vi "Lookup by Capabilities.vi"(8 "error in (no error)":errorcluster, 10 "Capabilities":string[](array[string]), 11 "NodeDiscovery in":refnum<class "DiscoveryService.lvclass">) -> (0 "error out":errorcluster, 2 "Nodes":T1[](array[typedef]), 3 "NodeDiscovery out":refnum<class "DiscoveryService.lvclass">)   [LabVIEW 2020, in "Vecto.lvlib" / "DiscoveryService.lvclass"]
uses:
  DiscoveryService.lvclass
  lv-volatus/messages/Discovery/Data.ctl
  lv-volatus/messages/Service/Data.ctl
  lv-volatus/messages/ServiceType/Enumeration.ctl
  lv-volatus/messages/ServiceType/ServiceType.lvlib
  lv-volatus/messages/Service/Service.lvlib
  lv-volatus/messages/Discovery/Discovery.lvlib
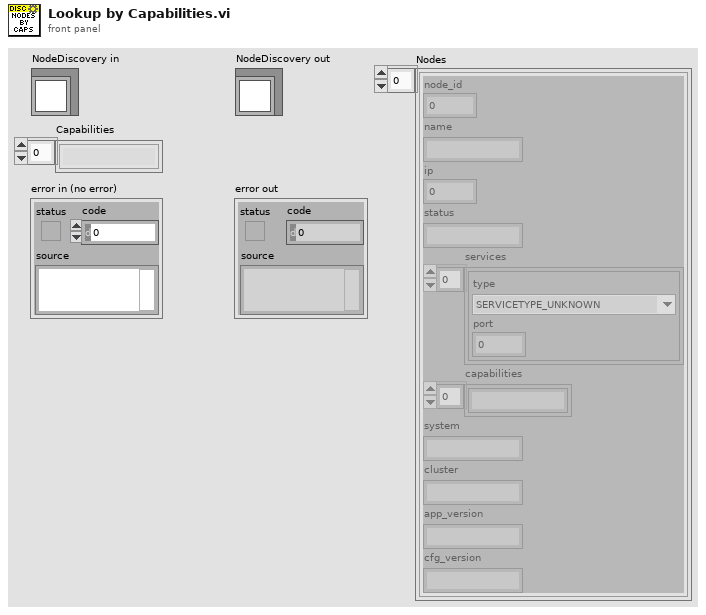
[diagram p1: front panel]
types:
  T1 = typedef "Discovery.lvlib/Data.ctl" = cluster{"node_id":u32, "name":string, "ip":u32, "status":string, "services":T2[], "capabilities":string[], "system":string, "cluster":string, "app_version":string, "cfg_version":string}
  T2 = typedef "Service.lvlib/Data.ctl" = cluster{"type":T3, "port":i32}
  T3 = typedef "ServiceType.lvlib/Enumeration.ctl" = enum16{"SERVICETYPE_UNKNOWN", "SERVICETYPE_TCPSERVER", "SERVICETYPE_HTTPSERVER"}
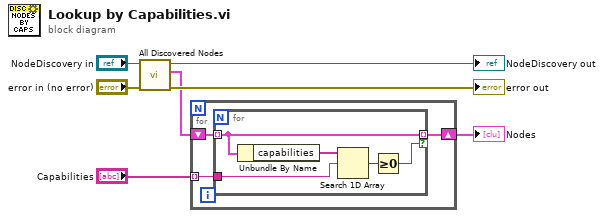
[diagram p0: block diagram]
diagram:
  n1 = call "All Discovered Nodes.vi"("error in (no error)"="error in (no error)", "DiscoveryService in"="NodeDiscovery in") -> ("error out"=→"error out":errorcluster, "Nodes"=w3:T1[], "DiscoveryService out"=→"NodeDiscovery out":refnum<class "DiscoveryService.lvclass">)  [unwired: 7 in]
  n2 = for {
    shift-right: [w8] -> w1
    shift-left: w3 -> [w10]
    tunnel: "Capabilities" -> [w9] mode=indexing
    n3 = for {
      tunnel: w10 -> [w12] mode=indexing
      tunnel: w9 -> [w14]
      tunnel: [w12] -> w8 mode=indexing if=w11
      n4 = Unbundle By Name(w12) -> ("capabilities"=w15:string[])
      n5 = Search 1D Array(1D array=w15, element=w14) -> (index of element=w13:i32)  [unwired: 1 in]
      n6 = Greater Or Equal To 0?(x=w13) -> (x >= 0?=w11:bool)
    }
  }
  "Nodes" <- w1
